vi "DisposeCore.vi"(8 "error in (no error)":errorcluster, 11 "ChicagoPizzaStore":refnum<class "ChicagoPizzaStore.lvclass">) -> (0 "error out":errorcluster, 3 "ChicagoPizzaStore":refnum<class "ChicagoPizzaStore.lvclass">)   [LabVIEW 2020, in "FactoryMethod.lvlib" / "PizzaFactoryMethod.lvlib" / "ChicagoPizzaStore.lvclass"]
uses:
  ChicagoPizzaStore.lvclass
  ChicagoPizzaStore.lvclass/ChicagoPizzaStore.ctl
  Private/TypeDef/privateDataDVR.ctl
  Private/TypeDef/privateData.ctl
  PizzaStore/PizzaStore.lvclass
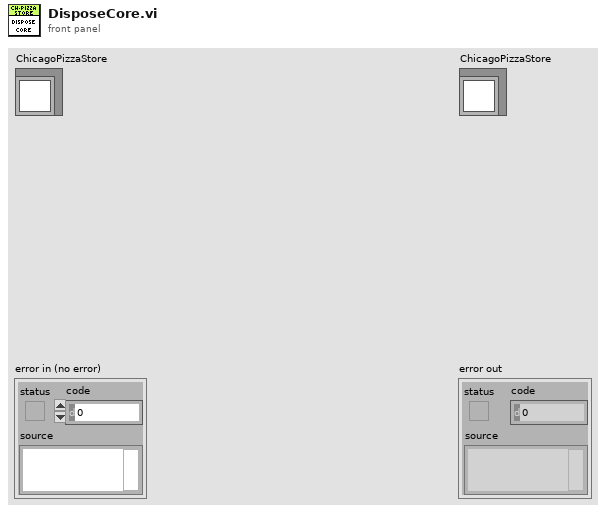
[diagram p1: front panel]
types:
  T1 = typedef "FactoryMethod.lvlib/PizzaFactoryMethod.lvlib/ChicagoPizzaStore.lvclass/privateDataDVR.ctl" = refnum<data-value>
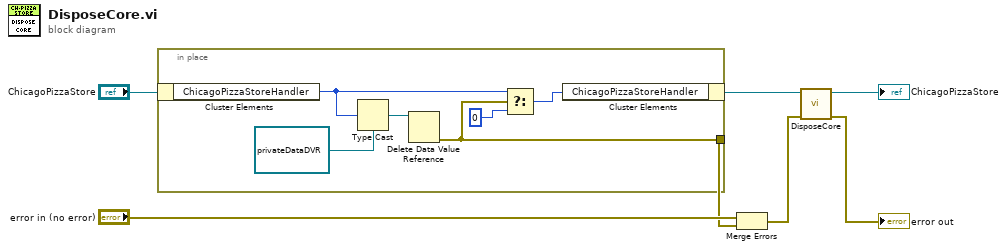
[diagram p0: block diagram]
diagram:
  n1 = in-place {
    in-place-border: [w12] -> w5
    n2 = in-place-cluster #1("ChicagoPizzaStore") -> ("ChicagoPizzaStoreHandler"=w11:u32)
    n3 = Type Cast(type=T1 refnum ("privateDataDVR"), x=w11) -> (*(type *) &x=w13:T1)
    n4 = Delete Data Value Reference(data value reference=w13) -> (error out=w12:errorcluster)  [unwired: 1 in, 1 out]
    n5 = Select(t=w11, s=w12, f=u32 0) -> (s? t:f=w10:u32)
    n6 = in-place-cluster #1("ChicagoPizzaStoreHandler"=w10) -> (w4:refnum<class "ChicagoPizzaStore.lvclass">)
  }
  n7 = Merge Errors("error in (no error)", w5) -> (w2:errorcluster)
  n8 = call-parent "DisposeCore.vi"("error in (no error)"=w2, "PizzaStore"=w4) -> ("error out"=→"error out":errorcluster, "PizzaStore"=→"ChicagoPizzaStore":refnum<class "ChicagoPizzaStore.lvclass">)  [unwired: 8 in]
